vi "GV_ToolbarSampleView.vi"(5 "Pixels":i32, 7 "Samples":i32, 8 "Hor-pos":i16, 9 "y":i16, 11 "Pict in":picture) -> (3 "Pict out":picture)   [LabVIEW 2020]
doc: "Andre Koelewijn, 30 June 2021\n\nDraw the number of samples in the toolbar"
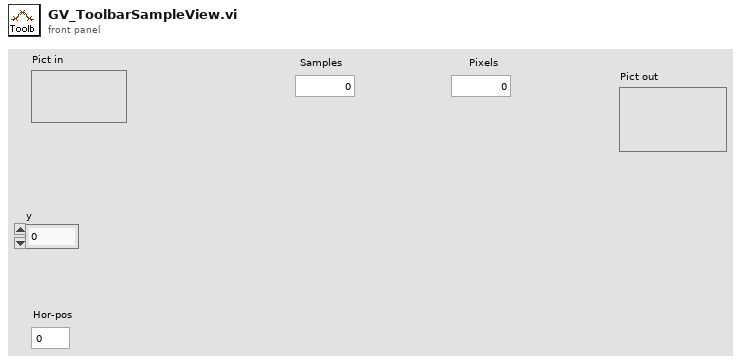
[diagram p1: front panel]
types:
  T1 = cluster{"horizontal":enum16{"left", "center", "right"}, "vertical":enum16{"top", "center", "bottom"}}
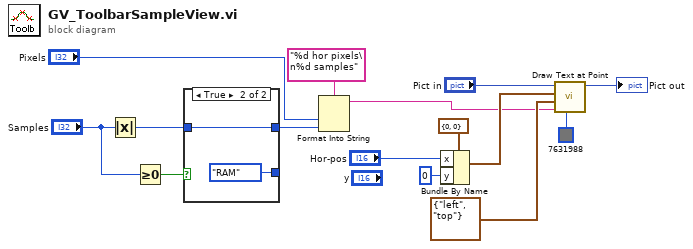
[diagram p0: block diagram]
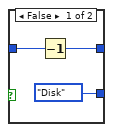
[diagram p2: hidden frame]
diagram:
  n1 = Absolute Value(x="Samples") -> (abs(x)=w9:i32)
  n2 = Greater Or Equal To 0?(x="Samples") -> (x >= 0?=w15:bool)
  n3 = case shown="True" w15 {
    tunnel: [enum16{"RAM", "Disk"}."Disk" ("MemoryType") enum16{"RAM", "Disk"}."RAM" ("MemoryType")] -> _
    tunnel: w9 -> [w17 w19]
    tunnel: [w16 w19] -> w5
    frame False {
      n4 = Decrement(x=w17) -> (x-1=w16:i32)
    }
    frame True {
    }
  }
  n5 = Format Into String(format string="%d hor pixels\n%d samples", "Pixels", w5) -> (resulting string=w3:string)  [unwired: 2 in, 1 out]
  n6 = Bundle By Name(cluster=cluster{"x":i16, "y":i16} {"x"=0, "y"=0} ("origin"), "x"="Hor-pos", "y"=i16 0) -> (w10:cluster{"x":i16, "y":i16})
  n7 = call <vilib>:"Draw Text at Point.vi"("text color(black)"=u32 7631988, "text"=w3, "alignment(left, top)"=T1 {"horizontal"=enum."left", "vertical"=enum."top"}, "origin"=w10, "picture"="Pict in") -> ("new picture"=→"Pict out":picture)  [unwired: 5 in, 1 out]
